vi "Material-ConfigDialog-UI.vi"(11 "error in":errorcluster) -> (15 "error out":errorcluster)   [LabVIEW 2014, in "Material-ConfigDialog.lvclass"]
uses:
  Material-ConfigDialog.lvclass
  Reuse Library/featherweight/Core/Sequencer/FTW-Sequencer.lvclass/FTW-Sequencer.ctl
  Material-ConfigDialog-Page.ctl
  Reuse Library/featherweight/Core/Messaging/Messenger.Actor/FTW-Messenger-Actor.lvclass
  Material-ConfigDialog.lvclass/Material-ConfigDialog.ctl
  <instrlib>/Keyence LK-G5000/Public/Constant/Comm Interface.ctl
  <vilib>/Utility/error.llb/DialogType.ctl
  Glue/Material-Glue-TreeItem.ctl
  Reuse Library/featherweight/Core/Regex/FTW-Regex.vi
  Reuse Library/featherweight/Core/Error/FTW-ERR-StatusException.vi
  Reuse Library/featherweight/Core/Error/FTW-ERR-ThrowError.vi
  Reuse Library/featherweight/Core/Error/FTW-ERR-Clear.vi
  Deploy Application/Material-Application-Constants.vi
  Reuse Library/featherweight/Core/Sequencer/FTW-Sequencer.lvclass
  Reuse Library/featherweight/Core/Messaging/Message.Actor/FTW-Message-Actor.lvclass
  Automation/Material-Automation-Website.ctl
  <instrlib>/Keyence LK-G5000/Keyence LK-G5000.lvlib
  <resource>/Framework/Providers/Wirebird Labs LLC/Deploy/Support/Update Service/Deploy-UpdateService.lvclass
panel:
  in  "UI_Tree_Navigation":string(tree) caption="Navigation Tree"
  in  "Hidden Controls\n(Tab Control Container)":enum32{"Just some hidden controls"}(tab)
  out "Status Bar Messages":string
  in  "UI-Button-Save":bool caption="Save Button"
  in  "UI-Button-Cancel":bool caption="Cancel Button"
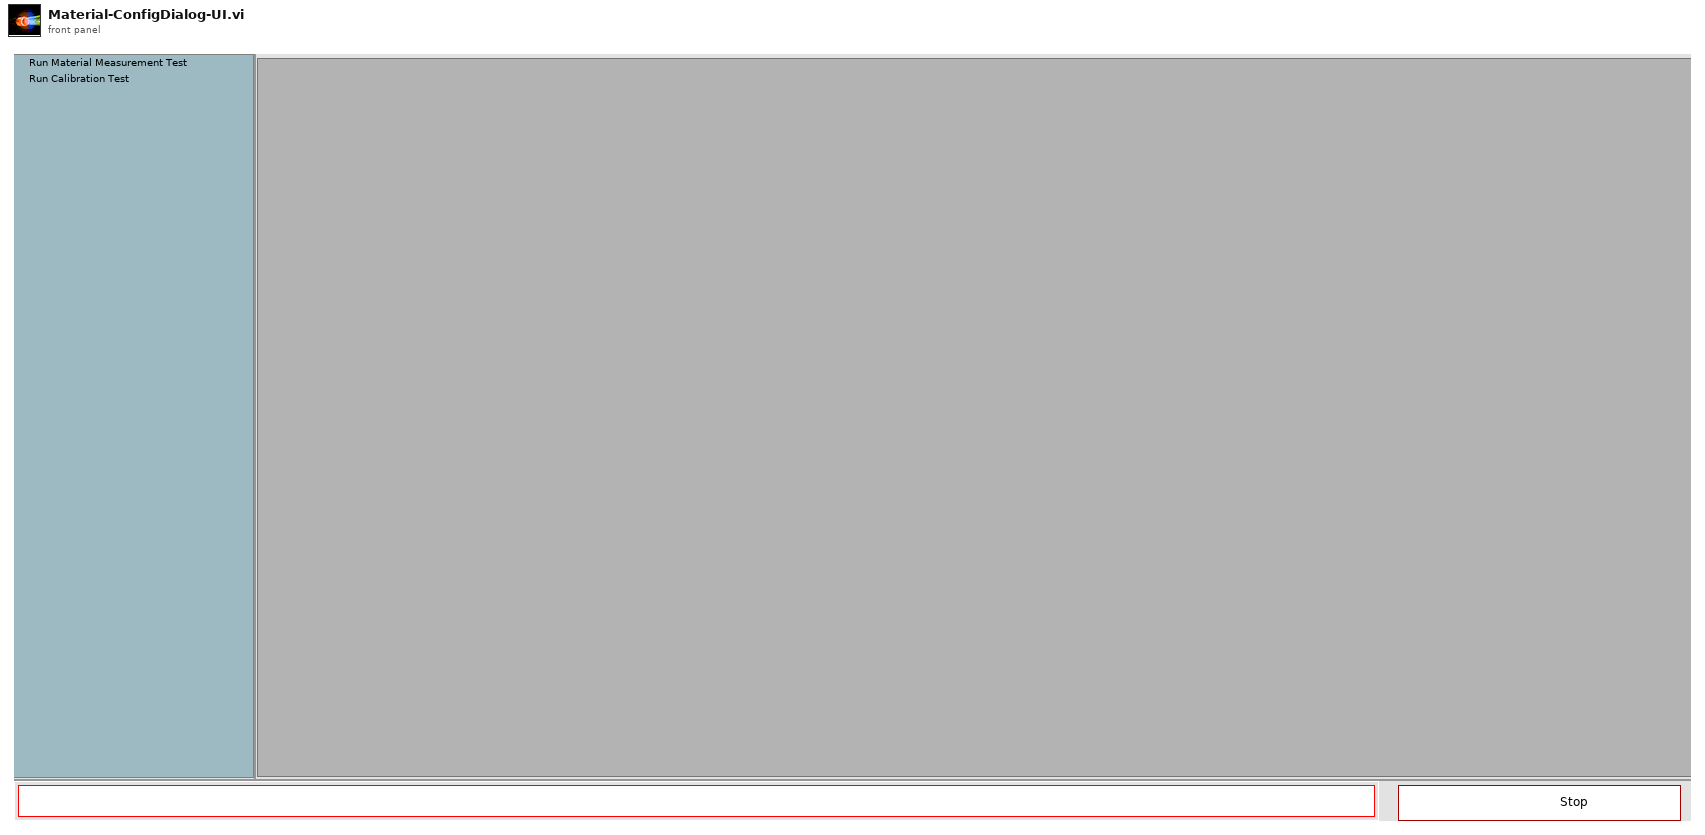
[diagram p1: front panel]
types:
  T1 = typedef "Material-Automation-Website.ctl" = enum16{"Wirebird Labs Home", "Wirebird Labs Support Home", "Wirebird Labs Licensing", "Wirebird Labs Idea Exchange", "Wirebird Labs Report a Bug", "Wirebird Labs Services Status", "Contact Wirebird Labs", "Deploy Documentation", "Deploy Credits", "Deploy Marketing", "Deploy Feature Matrix", "Deploy Purchase", "Deploy Deployment Servers"}
  T2 = typedef "Keyence LK-G5000.lvlib/Comm Interface.ctl" = enum8{"USB", "ETHERNET"}
  T3 = typedef "Material-Glue-TreeItem.ctl" = cluster{"Tag":string, "Parent":string, "Add to Top of Parent":bool, "Type":string, "Indent":i32, "Child Only":bool, "First Cell":string, "Next Cells":string[]}
  T4 = typedef "Material-ConfigDialog.lvclass/Material-ConfigDialog-Page.ctl" = cluster{"Initialized?":bool, "PageID":string, "Messenger":refnum<class "FTW-Messenger-Actor.lvclass">}
  T5 = cluster{"Configuration Dialog Mailbox":refnum<event-registration>, "Update Service Event Registration":refnum<event-registration>}
  T6 = typedef "DialogType.ctl" = u16
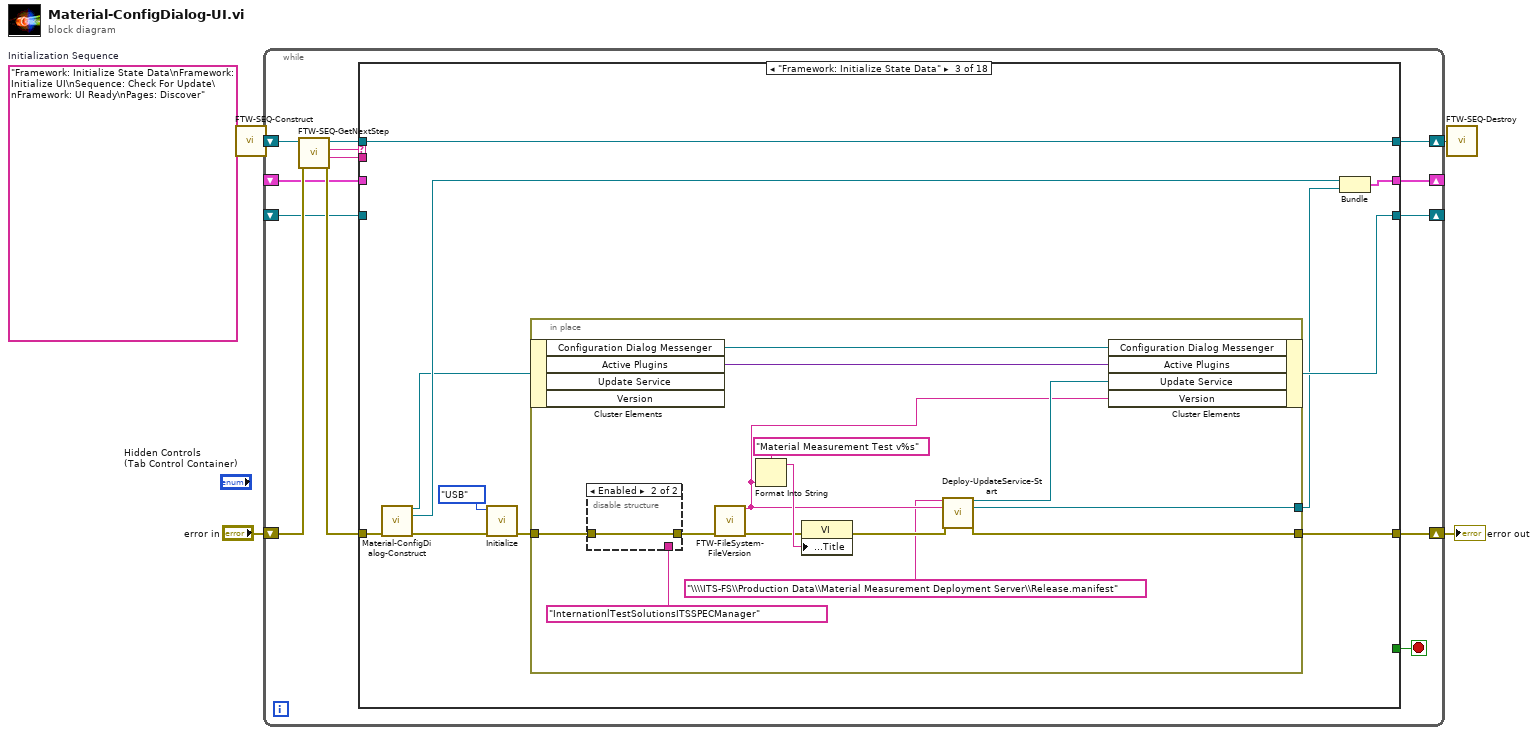
[diagram p0: block diagram]
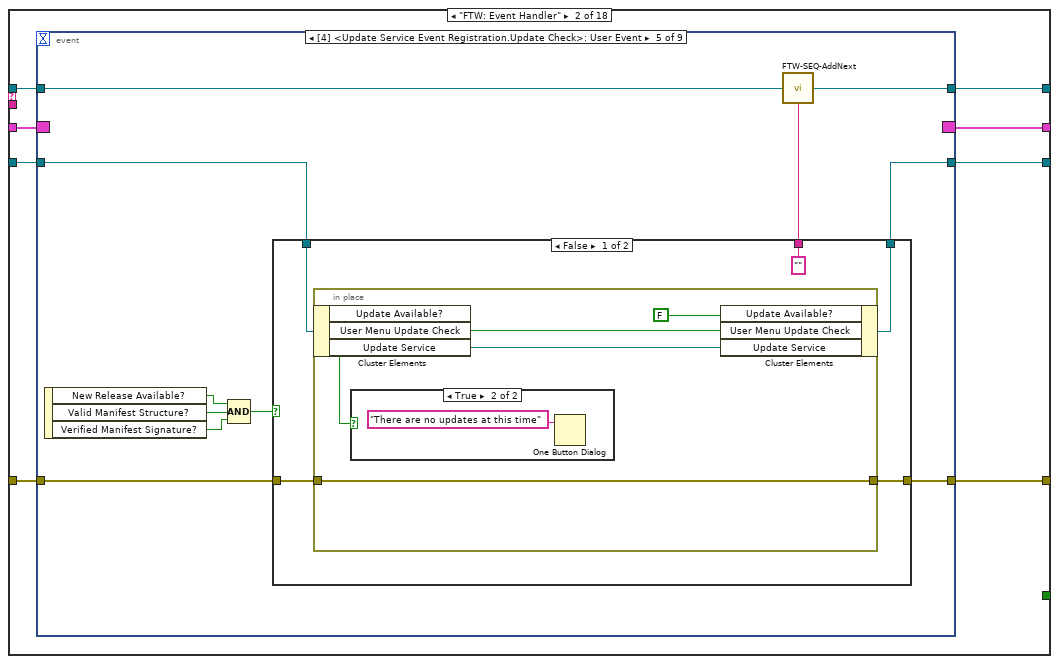
[diagram p3: hidden frame]
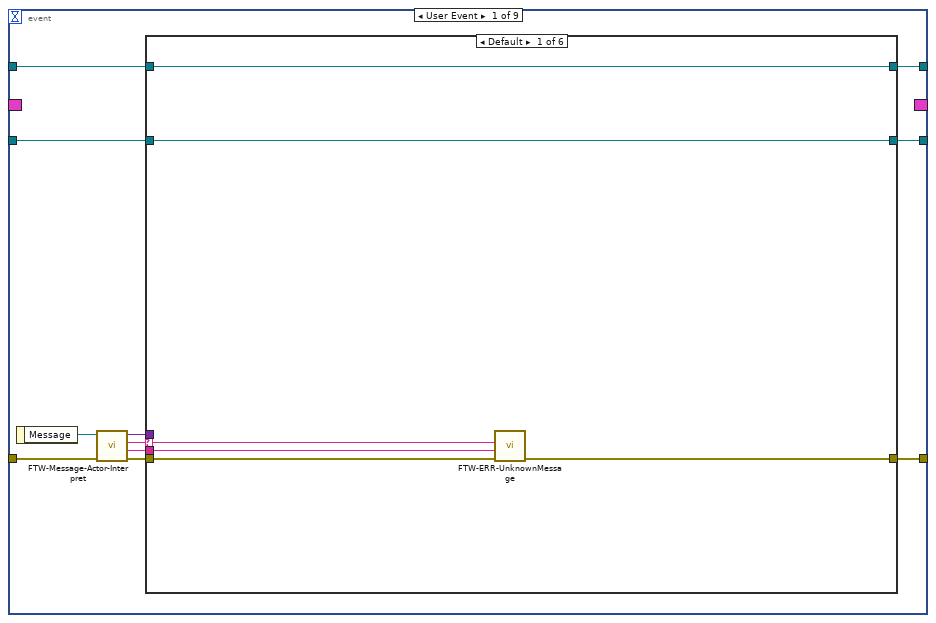
[diagram p4: hidden frame]
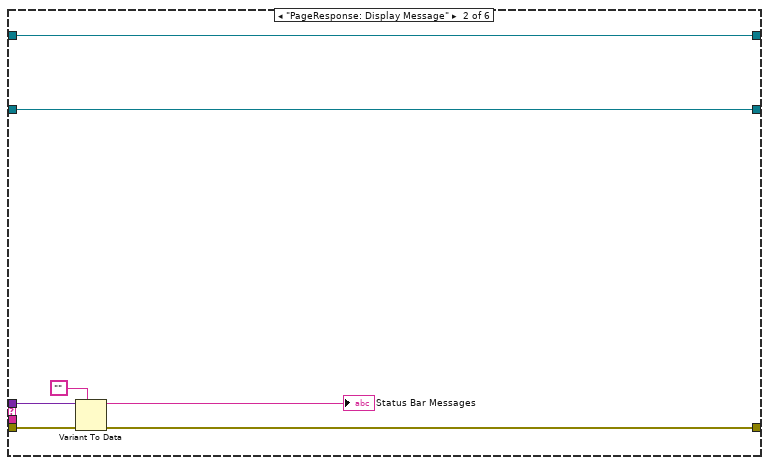
[diagram p5: hidden frame]
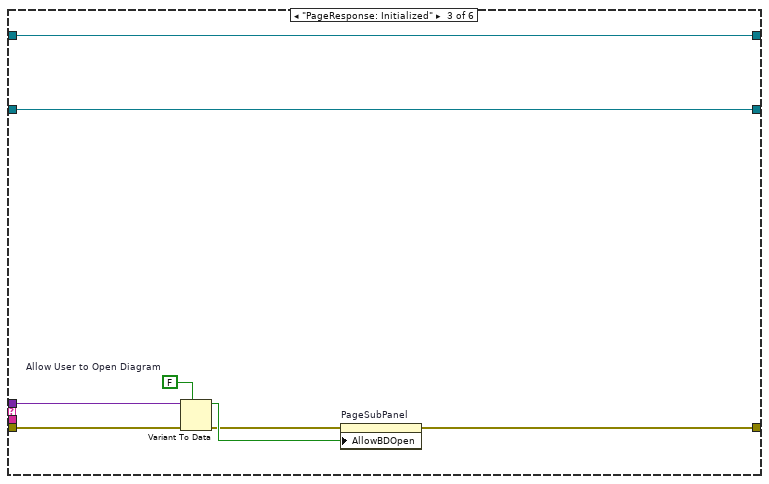
[diagram p6: hidden frame]
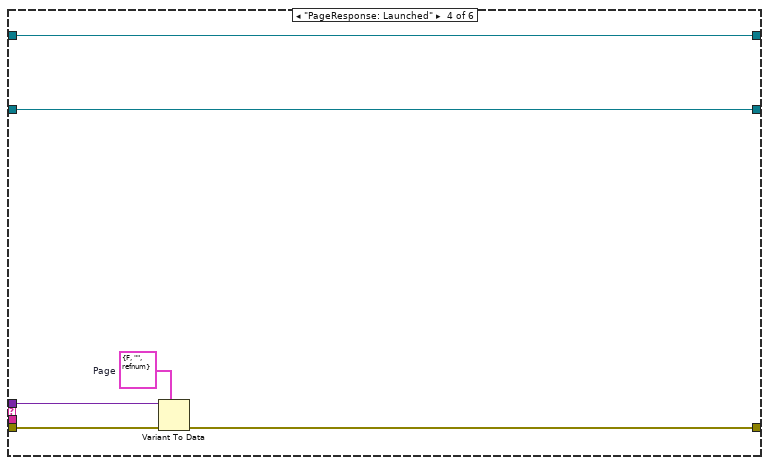
[diagram p7: hidden frame]
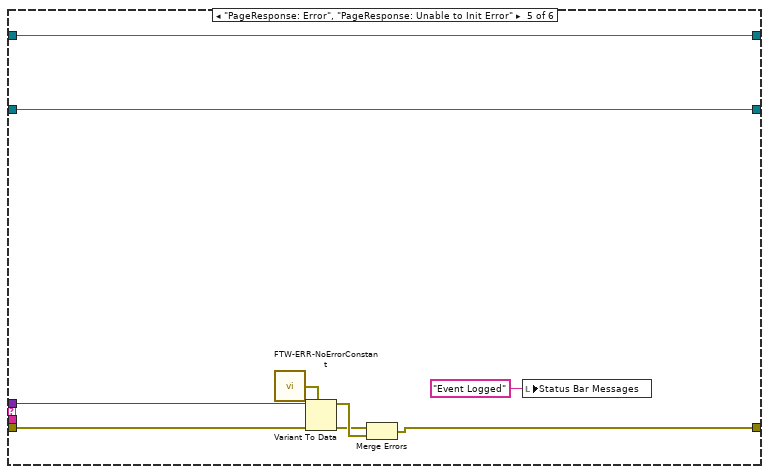
[diagram p8: hidden frame]
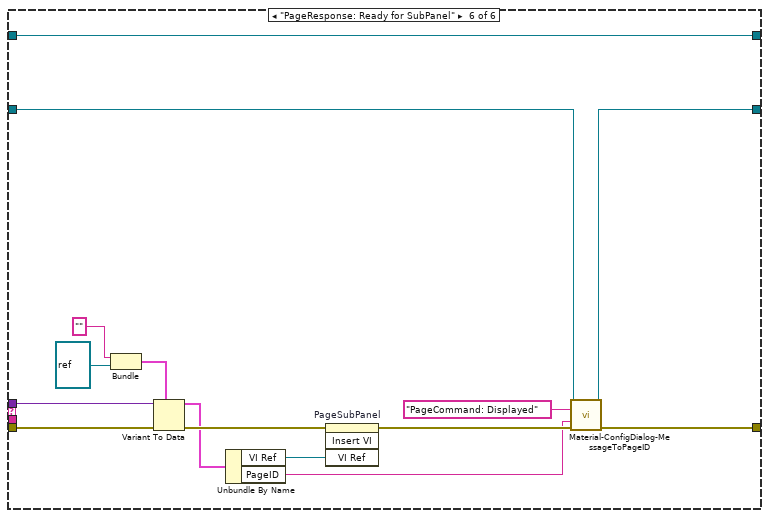
[diagram p9: hidden frame]
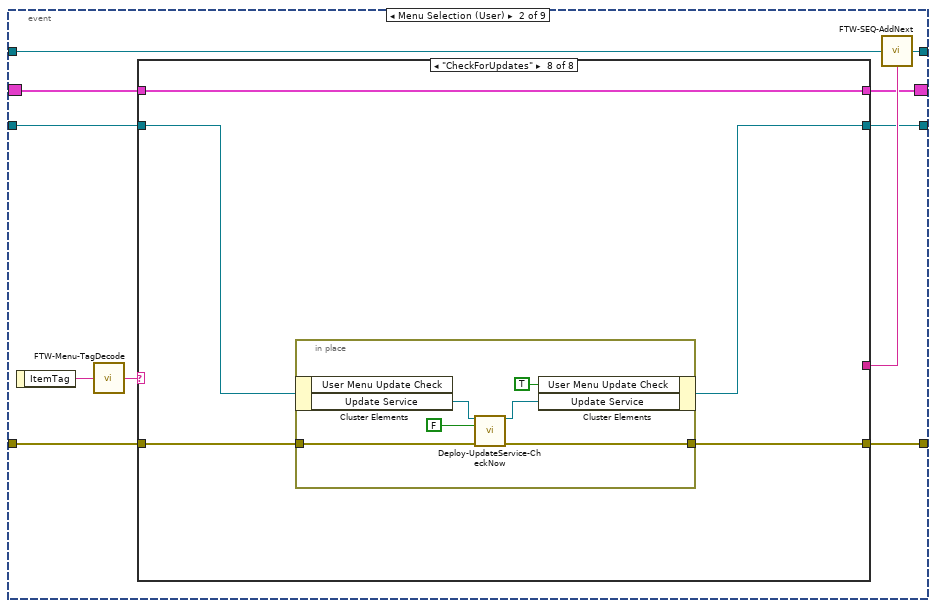
[diagram p10: hidden frame]
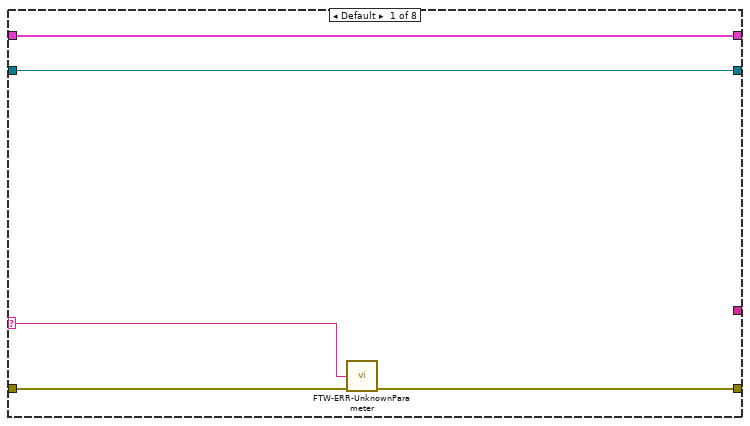
[diagram p11: hidden frame]
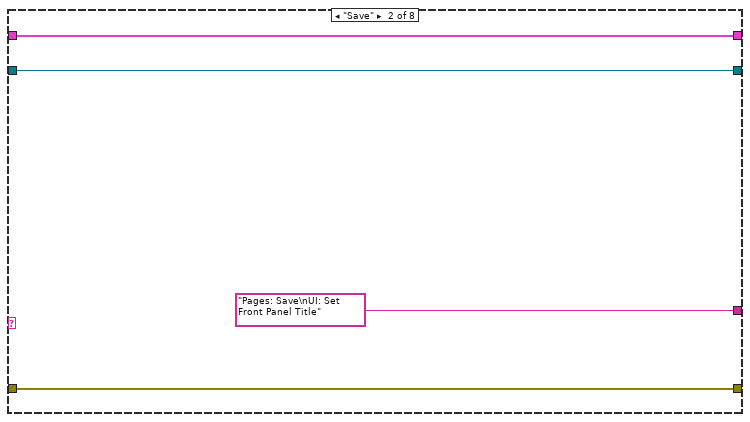
[diagram p12: hidden frame]
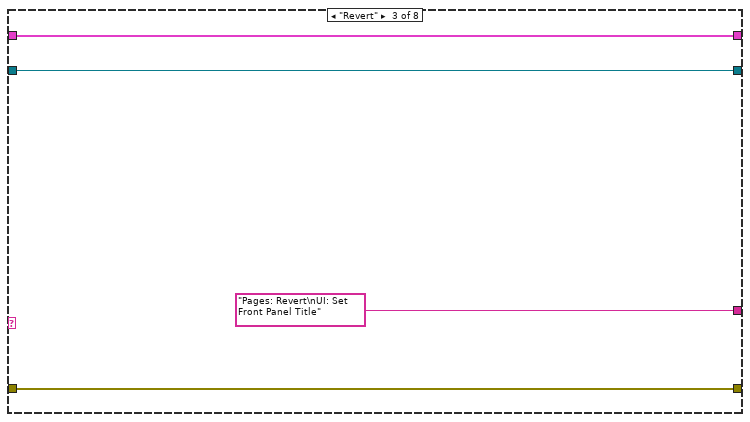
[diagram p13: hidden frame]
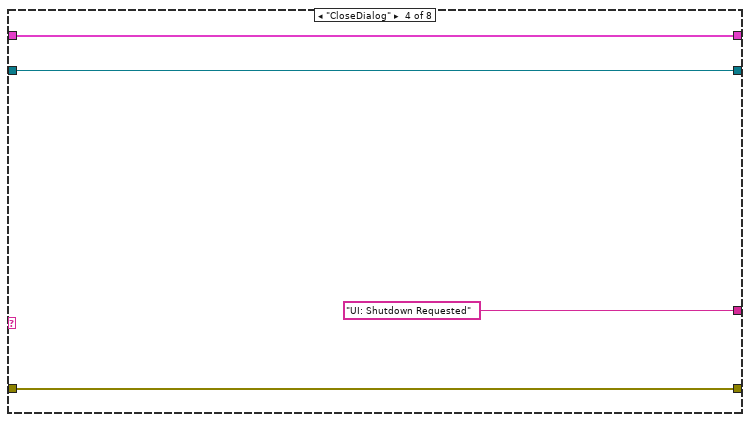
[diagram p14: hidden frame]
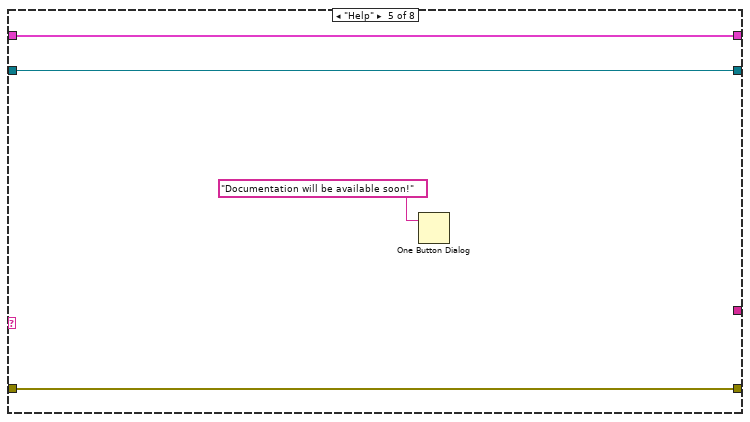
[diagram p15: hidden frame]
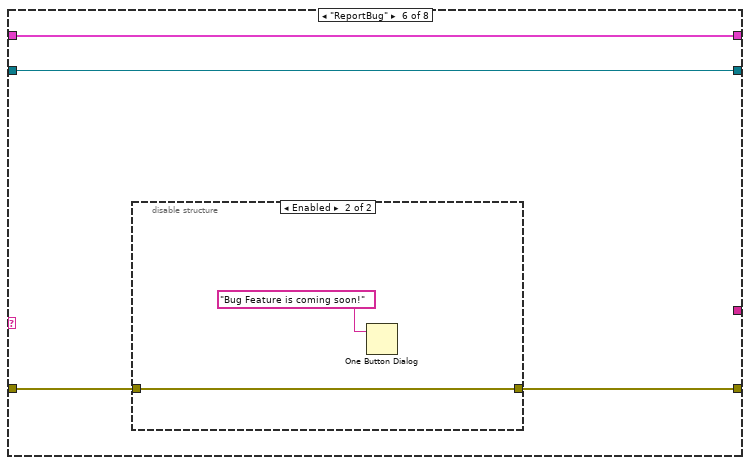
[diagram p16: hidden frame]
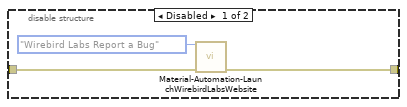
[diagram p17: hidden frame]
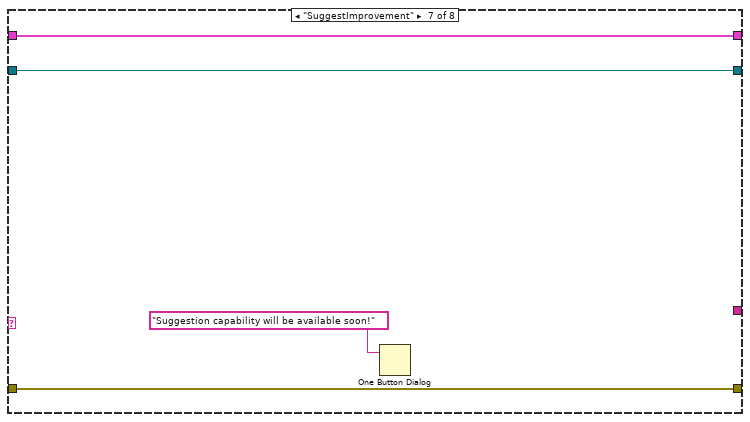
[diagram p18: hidden frame]
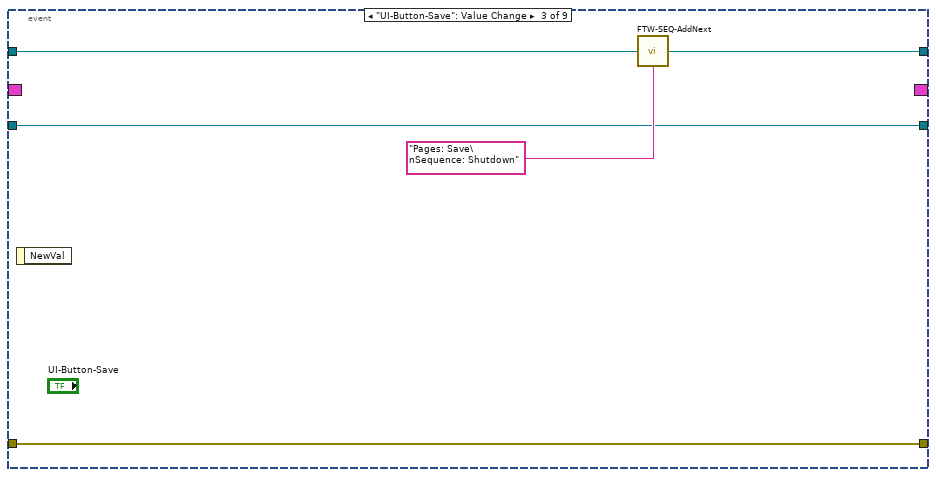
[diagram p19: hidden frame]
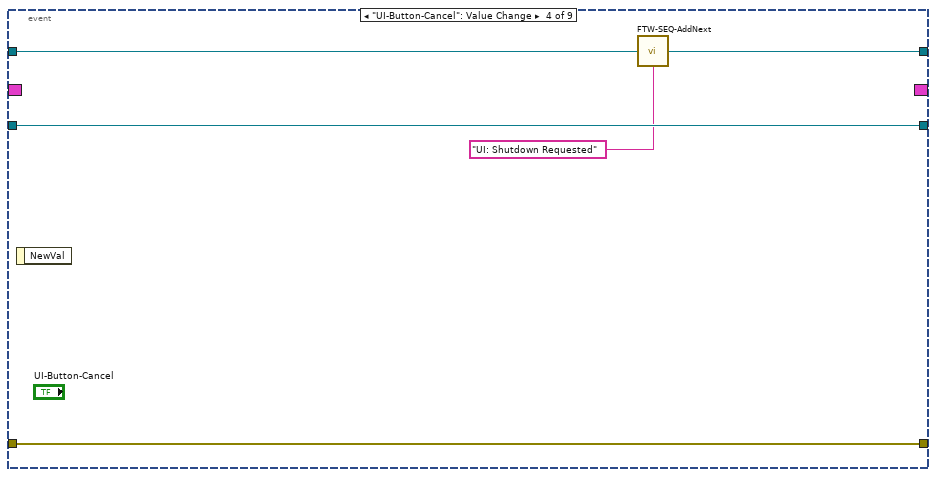
[diagram p20: hidden frame]
diagram:
  w5 = "Framework: Initialize State Data\nFramework: Initialize UI\nSequence: Check For Update\nFramework: UI Ready\nPages: Discover"  # Initialization Sequence
  n1 = call "FTW-SEQ-Construct.vi"("Initial Sequence"=w5) -> ("Sequencer"=w2:refnum<class "FTW-Sequencer.lvclass">)
  n2 = while {
    shift-right: [w16] -> w1
    shift-left: w2 -> [w7]
    shift-right: [w17] -> w4
    shift-left: "error in" -> [w15]
    shift-right: [w10] -> _
    shift-left: _ -> [w11]
    shift-right: [w9] -> _
    shift-left: _ -> [w8]
    stop <- w12 stop-if-true
    n3 = call "FTW-SEQ-GetNextStep.vi"("error in"=w15, "Sequencer"=w7) -> ("error out"=w18:errorcluster, "Job Data"=w6:string, "Current Job"=w13:string, "Sequencer out"=w14:refnum<class "FTW-Sequencer.lvclass">)  [unwired: 6 in]
    n4 = case shown="\"Framework: Initialize State Data\"" w13 {
      selector: w13 -> [_ _ _ _ _ _ w330 _ _ _ _ _ _ _ _ _ _ _]
      tunnel: [w20 w28 w258 w294 w318 w326 w332 w352 w353 w361 w367 w372 w393 w395 w411 w432 w445 w454] -> w17
      tunnel: w18 -> [w20 w27 w262 w295 w319 w324 w333 w348 w354 w361 w367 w373 w393 w395 w411 w420 w441 w449]
      tunnel: w14 -> [w22 w30 w261 w316 w322 w329 w335 w351 w359 w363 w364 w374 w392 w399 w412 w435 w448 w456]
      tunnel: [w22 w29 w261 w316 w322 w329 w335 w351 w359 w363 w369 w374 w392 w401 w412 w435 w448 w456] -> w16
      tunnel: [_ _ _ _ _ _ _ _ TRUE _ _ _ _ _ _ _ _ _] -> w12
      tunnel: w11 -> [w21 w25 _ w315 w321 w328 w334 w346 w357 w362 w368 w375 w394 w402 w414 w434 w447 w455]
      tunnel: [w21 w26 w263 w315 w321 w328 w334 w346 w357 w362 w368 w375 w394 w402 w414 w434 w447 w455] -> w10
      tunnel: [w19 w24 w257 w314 w320 w327 w331 w337 w356 w360 w365 w370 w391 w400 w413 w421 w446 w453] -> w9
      tunnel: w8 -> [w19 w23 _ w314 w320 w327 w331 w337 w356 w360 w365 w371 w391 w400 w413 w421 w442 w450]
      tunnel: w6 -> [_ _ _ _ _ _ _ _ _ _ _ _ _ _ _ _ _ _]
      frame "--------- Framework ---------" {
      }
      frame "FTW: Event Handler" {
        n5 = event shown="[4] <Update Service Event Registration.Update Check>: User Event" {
          selector: w25 -> [_ w93 _ _ _ _ _ _ _]
          dyn-events: [_ w94 _ _ _ _ _ _ _] -> w26
          timeout: _ -> [_ _ _ _ _ _ _ _ _]
          tunnel: w30 -> [w34 w99 w149 w155 w161 w204 w222 w244 w248]
          tunnel: [w35 w103 w153 w158 w163 w204 w222 w244 w251] -> w29
          tunnel: [w38 w100 w152 w156 w160 w209 w223 w245 w252] -> w28
          tunnel: w27 -> [w39 w101 w152 w156 w159 w210 w219 w246 w252]
          tunnel: [w37 w96 w150 w157 w164 w205 w221 w243 w249] -> w24
          tunnel: w23 -> [w36 w95 w150 w157 w165 w205 w216 w243 w249]
          event User Event {
            n6 = event-data() -> ("Message"=w40:refnum<class "FTW-Message.lvclass">)  [unwired: 1 in]
            n7 = call "FTW-Message-Actor-Interpret.vi"("error in"=w39, "Message"=w40) -> ("error out"=w41:errorcluster, "Sender"=w31:string, "Parameter"=w33:string, "Payload"=w32:variant)  [unwired: 6 in]
            n8 = case shown="Default" w33 {
              selector: w33 -> [w43 _ _ _ _ _]
              tunnel: w32 -> [_ w54 w55 w65 w77 w92]
              tunnel: [w46 w52 w56 w63 w69 w85] -> w38
              tunnel: w41 -> [w47 w53 w60 w64 w76 w91]
              tunnel: [w44 w48 w62 w68 w73 w87] -> w37
              tunnel: w36 -> [w44 w48 w62 w68 w73 w88]
              tunnel: [w45 w49 w61 w67 w74 w90] -> w35
              tunnel: w34 -> [w45 w49 w61 w67 w74 w90]
              tunnel: w31 -> [w42 _ _ _ _ _]
              frame Default {
                n9 = call "FTW-ERR-UnknownMessage.vi"("error in"=w47, "Sender"=w42, "Unknown Parameter"=w43) -> ("error out"=w46:errorcluster)  [unwired: 8 in]
              }
              frame "PageResponse: Display Message" {
                n10 = Variant To Data(error in=w53, type="", Variant=w54) -> (data=→"Status Bar Messages":string, error out=w52:errorcluster)
              }
              frame "PageResponse: Initialized" {
                w59 = FALSE  # Allow User to Open Diagram
                n11 = Variant To Data(error in=w60, type=w59, Variant=w55) -> (data=w58:bool, error out=w57:errorcluster)
                n12 = property on="PageSubPanel" class="SubPnl"(error in=w57, "AllowBDOpen"=w58) -> (error out=w56:errorcluster)  [unwired: 1 in, 1 out]
              }
              frame "PageResponse: Launched" {
                w66 = T4 {"Initialized?"=FALSE, "PageID"="", "Messenger"=refnum}  # Page
                n13 = Variant To Data(error in=w64, type=w66, Variant=w65) -> (error out=w63:errorcluster)  [unwired: 1 out]
              }
              frame "PageResponse: Error", "PageResponse: Unable to Init Error" {
                n14 = call "FTW-ERR-NoErrorConstant.vi"() -> ("no error"=w75:errorcluster)
                n15 = Variant To Data(error in=w76, type=w75, Variant=w77) -> (data=w71:errorcluster, error out=w70:errorcluster)
                n16 = Merge Errors(w70, w71) -> (w69:errorcluster)
                n17 = local write "Status Bar Messages"("Event Logged" ("Status Bar Messages")) -> ()
              }
              frame "PageResponse: Ready for SubPanel" {
                n18 = Bundle("PageID"="", "VI Ref"=refnum<vi> refnum) -> (w81:cluster{"PageID":string, "VI Ref":refnum<vi>})  [unwired: 1 in]
                n19 = Variant To Data(error in=w91, type=w81, Variant=w92) -> (data=w80:cluster{"PageID":string, "VI Ref":refnum<vi>}, error out=w84:errorcluster)
                n20 = Unbundle By Name(w80) -> ("VI Ref"=w79:refnum<vi>, "PageID"=w78:string)
                n21 = invoke on="PageSubPanel" class="SubPanel" method="Insert VI"(error in=w84, "VI Ref"=w79) -> (error out=w86:errorcluster)  [unwired: 2 in, 3 out]
                n22 = call "Material-ConfigDialog-MessageToPageID.vi"("Configuration Dialog"=w88, "Parameter"="PageCommand: Displayed", "PageID"=w78, "error in"=w86) -> ("Configuration Dialog out"=w87:refnum<class "Material-ConfigDialog.lvclass">, "error out"=w85:errorcluster)  [unwired: 10 in]
              }
            }
          }
          event Menu Selection (User) {
            n23 = event-data() -> ("ItemTag"=w98:string)  [unwired: 1 in]
            n24 = call "FTW-Menu-TagDecode.vi"("Menu Item Tag"=w98) -> ("Command"=w97:string)  [unwired: 1 in, 2 out]
            n25 = case shown="\"CheckForUpdates\"" w97 {
              selector: w97 -> [w105 _ _ _ _ _ _ _]
              tunnel: [_ "Pages: Save\nUI: Set Front Panel Title" ("Add to Top of Queue") "Pages: Revert\nUI: Set Front Panel Title" ("Add to Top of Queue") "UI: Shutdown Requested" ("Add to Top of Queue") _ _ _ _] -> w102
              tunnel: w101 -> [w108 w111 w115 w119 w124 w128 w135 w141]
              tunnel: [w107 w111 w115 w119 w124 w127 w135 w140] -> w100
              tunnel: [w106 w110 w114 w118 w123 w126 w137 w138] -> w96
              tunnel: w95 -> [w106 w110 w114 w118 w123 w126 w137 w139]
              tunnel: [w104 w109 w113 w117 w122 w125 w136 w142] -> w94
              tunnel: w93 -> [w104 w109 w113 w117 w122 w125 w136 w142]
              frame Default {
                n26 = call "FTW-ERR-UnknownParameter.vi"("Unknown Parameter"=w105, "error in"=w108) -> ("error out"=w107:errorcluster)  [unwired: 13 in]
              }
              frame "Save" {
              }
              frame "Revert" {
              }
              frame "CloseDialog" {
              }
              frame "Help" {
                n27 = One Button Dialog(message="Documentation will be available soon!") -> ()  [unwired: 1 in, 1 out]
              }
              frame "ReportBug" {
                n28 = disable-structure shown="Enabled" {
                  disable-tunnel: w128 -> [w131 w133]
                  disable-tunnel: [w130 w133] -> w127
                  frame Disabled {
                    n29 = call "Material-Automation-LaunchWirebirdLabsWebsite.vi"("Site to Launch"=Material-Automation-Website."Wirebird Labs Report a Bug", "error in"=w131) -> ("error out"=w130:errorcluster)  [unwired: 13 in]
                  }
                  frame Enabled {
                    n30 = One Button Dialog(message="Bug Feature is coming soon!") -> ()  [unwired: 1 in, 1 out]
                  }
                }
              }
              frame "SuggestImprovement" {
                n31 = One Button Dialog(message="Suggestion capability will be available soon!") -> ()  [unwired: 1 in, 1 out]
              }
              frame "CheckForUpdates" {
                n32 = in-place {
                  in-place-border: w141 -> [w148]
                  in-place-border: [w144] -> w140
                  n33 = in-place-cluster #1(w139) -> ("Update Service"=w146:refnum<class "Deploy-UpdateService.lvclass">)  [unwired: 1 out]
                  n34 = call <resource>:"Deploy-UpdateService-CheckNow.vi"("Update Service"=w146, "Show UI?"=FALSE, "error in"=w148) -> ("Update Service out"=w145:refnum<class "Deploy-UpdateService.lvclass">, "error out"=w144:errorcluster)  [unwired: 11 in]
                  n35 = in-place-cluster #1("User Menu Update Check"=TRUE, "Update Service"=w145) -> (w138:refnum<class "Material-ConfigDialog.lvclass">)
                }
              }
            }
            n36 = call "FTW-SEQ-AddNext.vi"("Add Next in Sequence"=w102, "Sequencer"=w99) -> ("Sequencer out"=w103:refnum<class "FTW-Sequencer.lvclass">)  [unwired: 2 in]
          }
          event "UI-Button-Save": Value Change {
            n37 = event-data() -> ()  [unwired: 1 in, 1 out]
            n38 = call "FTW-SEQ-AddNext.vi"("Add Next in Sequence"="Pages: Save\nSequence: Shutdown" ("Add to Top of Queue"), "Sequencer"=w149) -> ("Sequencer out"=w153:refnum<class "FTW-Sequencer.lvclass">)  [unwired: 2 in]
          }
          event "UI-Button-Cancel": Value Change {
            n39 = event-data() -> ()  [unwired: 1 in, 1 out]
            n40 = call "FTW-SEQ-AddNext.vi"("Add Next in Sequence"="UI: Shutdown Requested" ("Add to Top of Queue"), "Sequencer"=w155) -> ("Sequencer out"=w158:refnum<class "FTW-Sequencer.lvclass">)  [unwired: 2 in]
          }
          event User Event {
            n41 = event-data() -> ("New Release Available?"=w169:bool, "Valid Manifest Structure?"=w168:bool, "Verified Manifest Signature?"=w167:bool)  [unwired: 1 in]
            n42 = Compound Arithmetic op=AND(w169, w168, w167) -> (w166:bool)
            n43 = case shown="False" w166 {
              selector: w166 -> [_ w182]
              tunnel: w159 -> [w172 w185]
              tunnel: w165 -> [w173 w183]
              tunnel: [w170 w181] -> w164
              tunnel: [w171 w184] -> w160
              tunnel: ["" ("Application Shutdown") w180] -> w162
              frame False {
                n44 = in-place {
                  in-place-border: w172 -> [w175]
                  in-place-border: [w175] -> w171
                  n45 = in-place-cluster #2(w173) -> ("User Menu Update Check"=w178:bool, "Update Service"=w176:refnum<class "Deploy-UpdateService.lvclass">)  [unwired: 1 out]
                  n46 = case shown="True" w178 {
                    frame False {
                    }
                    frame True {
                      n47 = One Button Dialog(message="There are no updates at this time" ("Application Shutdown")) -> ()  [unwired: 1 in, 1 out]
                    }
                  }
                  n48 = in-place-cluster #2("Update Available?"=FALSE, "User Menu Update Check"=w178, "Update Service"=w176) -> (w170:refnum<class "Material-ConfigDialog.lvclass">)
                }
              }
              frame True {
                n49 = in-place {
                  in-place-border: w185 -> [w195]
                  in-place-border: [w190] -> w184
                  in-place-border: w182 -> [_]
                  in-place-border: [w186] -> w180
                  n50 = in-place-cluster #3(w183) -> ("Update Service"=w194:refnum<class "Deploy-UpdateService.lvclass">, "Version"=w188:string)  [unwired: 1 out]
                  n51 = call <resource>:"Deploy-UpdateService-Stop.vi"("Update Service"=w194, "error in"=w195) -> ("error out"=w192:errorcluster)  [unwired: 13 in]
                  n52 = Equal?(x=w188, y="IDE") -> (x = y?=w189:bool)
                  n53 = case shown="True" w189 {
                    tunnel: w192 -> [w201 w203]
                    tunnel: "\\\\ITS-FS\\Production Data\\Material Measurement Deployment Server\\Release.manifest" ("Manifest URI") -> [w200 _]
                    tunnel: [w198 w203] -> w190
                    tunnel: w188 -> [w197 _]
                    tunnel: [w196 "" ("Application Shutdown")] -> w186
                    frame False {
                      w196 = "Sequence: Shutdown"  # Application Shutdown
                      n54 = call <resource>:"Deploy-UpdateService-LaunchUI-Async.vi"("Manifest URI"=w200, "Current Release Version"=w197, "error in"=w201, "Installer Command Line Parameters"="") -> ("error out"=w198:errorcluster)  [unwired: 10 in, 1 out]
                    }
                    frame True {
                    }
                  }
                  n55 = in-place-cluster #3("Update Service"=w194, "Update Available?"=TRUE ("Boolean"), "Version"=w188) -> (w181:refnum<class "Material-ConfigDialog.lvclass">)
                }
              }
            }
            n56 = call "FTW-SEQ-AddNext.vi"("Add Next in Sequence"=w162, "Sequencer"=w161) -> ("Sequencer out"=w163:refnum<class "FTW-Sequencer.lvclass">)  [unwired: 2 in]
          }
          event User Event {
            n57 = event-data() -> ("Error Status"=w208:bool, "Error Code"=w207:i32, "Error Message"=w206:string)  [unwired: 1 in]
            n58 = Format Into String(format string="Uh-oh! Something went wrong! This is what happened:\n\nError %d: \"%s\"", w207, w206) -> (resulting string=w212:string)  [unwired: 2 in, 1 out]
            n59 = One Button Dialog(message=w212) -> ()  [unwired: 1 in, 1 out]
            n60 = Bundle By Name(cluster=w210, "status"=w208, "code"=w207, "source"=w206) -> (w209:errorcluster)
          }
          event "UI_Tree_Navigation": Value Change {
            n61 = event-data() -> ("NewVal"=w214:string)  [unwired: 1 in]
            n62 = call "FTW-Menu-TagDecode.vi"("Menu Item Tag"=w214) -> ("Command"=w220:string, "Payload"=w217:string)  [unwired: 1 in, 1 out]
            n63 = case shown="\"UninitializedPage\"" w220 {
              tunnel: w219 -> [w227 w231 w242]
              tunnel: [w226 w231 w233] -> w218
              tunnel: w217 -> [_ _ w241]
              tunnel: w216 -> [w225 w230 w239]
              tunnel: [w225 w230 w238] -> w215
              tunnel: w214 -> [_ _ w236]
              tunnel: [_ "UI_Tree_Navigation" w235] -> w213
              frame Default {
                n64 = call "FTW-ERR-ThrowGenericError.vi"("Error Message"="Unknown Navigation Tree item.", "error in"=w227) -> ("error out"=w226:errorcluster)  [unwired: 13 in]
              }
              frame "ActivePage" {
                # "Already launched; just notify it\nneeds to get ready for SubPanel"
              }
              frame "UninitializedPage" {
                # "Keep\nselection"
                n65 = String To Path(string=w241) -> (path=w240:path)
                n66 = call "Material-ConfigDialog-LaunchPage.vi"("Configuration Dialog"=w239, "Configuration Page VI Filepath"=w240, "error in"=w242) -> ("Configuration Dialog out"=w238:refnum<class "Material-ConfigDialog.lvclass">, "New Navigation Tree Tag"=w235:string, "error out"=w237:errorcluster)  [unwired: 9 in, 1 out]
                n67 = invoke on="UI_Tree_Navigation" class="Tree (strict)" method="Edit Tree Items.Set Tag"(error in=w237, "tag"=w236, "new tag"=w235) -> (error out=w234:errorcluster, "Edit Tree Items:Set Tag"=w232:string)  [unwired: 2 in, 3 out]
                n68 = property on="UI_Tree_Navigation" class="Tree (strict)"(error in=w234, "Value"=w232) -> (error out=w233:errorcluster)  [unwired: 1 in, 1 out]
              }
            }
            n69 = call "Material-ConfigDialog-MessageToPageID.vi"("Configuration Dialog"=w215, "Parameter"="PageCommand: Prepare for SubPanel", "PageID"=w213, "error in"=w218) -> ("Configuration Dialog out"=w221:refnum<class "Material-ConfigDialog.lvclass">, "error out"=w223:errorcluster)  [unwired: 10 in]
          }
          event "UI_Tree_Navigation": Mouse Down {
            # "Just ensure the pesky dotted box\nsurrounding the item does not show up"
            n70 = event-data() -> ()  [unwired: 1 in, 2 out]
            n71 = property on="UI_Tree_Navigation" class="Tree (strict)"(error in=w246, "Key Focus"=FALSE) -> (error out=w245:errorcluster)  [unwired: 1 in, 1 out]
          }
          event Panel Close? {
            n72 = event-data() -> ()  [unwired: 1 in, 1 out]
            n73 = call "FTW-SEQ-AddNext.vi"("Add Next in Sequence"="UI: Shutdown Requested" ("Add to Top of Queue"), "Sequencer"=w248) -> ("Sequencer out"=w251:refnum<class "FTW-Sequencer.lvclass">)  [unwired: 2 in]
            n74 = event-data("Discard?"=TRUE) -> ()  [unwired: 1 in, 1 out]
          }
        }
      }
      frame "Framework: Initialize State Data" {
        n75 = call "Material-ConfigDialog-Construct.vi"("error in"=w262) -> ("Configuration Dialog"=w259:refnum<class "Material-ConfigDialog.lvclass">, "Configuration Dialog Mailbox"=w264:refnum<event-registration>, "error out"=w255:errorcluster)  [unwired: 12 in]
        n76 = call <instrlib>:"Initialize.vi"("error in (no error)"=w255, "Comm Interface"=Comm_Interface."USB") -> ("error out"=w254:errorcluster)  [unwired: 9 in]
        n77 = in-place {
          in-place-border: [w278] -> w256
          in-place-border: [w274] -> w258
          in-place-border: w254 -> [w265]
          n78 = in-place-cluster #4(w259) -> ("Configuration Dialog Messenger"=w275:refnum<class "FTW-Messenger-Actor.lvclass">, "Active Plugins"=w276:variant)  [unwired: 2 out]
          n79 = disable-structure shown="Enabled" {
            disable-tunnel: w265 -> [w281 w282]
            disable-tunnel: [w280 w282] -> w269
            disable-tunnel: "InternationlTestSolutionsITSSPECManager" ("format string") -> [w279 _]
            frame Disabled {
              n80 = call <resource>:"Deploy-Update-CreateAppMutex.vi"("Application Mutex Name"=w279, "error in"=w281) -> ("error out"=w280:errorcluster)  [unwired: 13 in]
            }
            frame Enabled {
            }
          }
          n81 = call "FTW-FileSystem-FileVersion.vi"("error in"=w269) -> ("Version"=w268:string, "error out"=w271:errorcluster)  [unwired: 13 in]
          n82 = Format Into String(format string="Material Measurement Test v%s", w268) -> (resulting string=w272:string)  [unwired: 2 in, 1 out]
          n83 = property class="VI"(error in=w271, "Front Panel.Title"=w272) -> (error out=w270:errorcluster)  [unwired: 1 in, 1 out]
          n84 = call <resource>:"Deploy-UpdateService-Start.vi"("Manifest URI"="\\\\ITS-FS\\Production Data\\Material Measurement Deployment Server\\Release.manifest", "Current Release Version"=w268, "error in"=w270) -> ("Update Service"=w277:refnum<class "Deploy-UpdateService.lvclass">, "Update Service Event Registration"=w278:refnum<event-registration>, "error out"=w274:errorcluster)  [unwired: 10 in]
          n85 = in-place-cluster #4("Configuration Dialog Messenger"=w275, "Active Plugins"=w276, "Update Service"=w277, "Version"=w268) -> (w257:refnum<class "Material-ConfigDialog.lvclass">)
        }
        n86 = Bundle("Configuration Dialog Mailbox"=w264, "Update Service Event Registration"=w256) -> (w263:T5)  [unwired: 1 in]
      }
      frame "Framework: Initialize UI" {
        w297 = i16 40 ("Vertical")
        w300 = i16 240 ("Horizontal")
        w306 = 2000  # Much wider than ever expected to be
        n87 = invoke on="UI_Tree_Navigation" class="Tree (strict)" method="Edit Tree Items.Delete"("Delete Children"=TRUE ("Delete Children?")) -> (error out=w291:errorcluster)  [unwired: 4 in, 4 out]
        n88 = call "Material-Application-MinimumPageSize.vi"("error in"=w295) -> ("Minimum Pane Size"=w290:cluster{"Horizontal":i16, "Vertical":i16}, "error out"=w305:errorcluster)  [unwired: 13 in]
        n89 = Bundle By Name(cluster=w290, "Horizontal"=w300) -> (w304:cluster{"Horizontal":i16, "Vertical":i16})
        n90 = Bundle By Name(cluster=w290, "Horizontal"=i16 310, "Vertical"=w297) -> (w303:cluster{"Horizontal":i16, "Vertical":i16})
        n91 = global read "Material-Application-Constants.vi" "Color.Selection"() -> (w287:u32)
        n92 = Add(x=cluster{"Horizontal":i16, "Vertical":i16} {"Horizontal"=24, "Vertical"=0}, y=w290) -> (x+y=w288:cluster{"Horizontal":i16, "Vertical":i16})
        n93 = Unbundle By Name(w288) -> ("Horizontal"=w301:i16, "Vertical"=w298:i16)
        n94 = property on="UserInterface-Pane-Page" class="Pane"(error in=w305, "Minimum Pane Size"=w288) -> (error out=w312:errorcluster)  [unwired: 1 in, 1 out]
        n95 = property on="UserInterface-Pane-Navigation" class="Pane"("Minimum Pane Size"=w304) -> (error out=w310:errorcluster)  [unwired: 2 in, 1 out]
        n96 = property on="UserInterface-Pane-Buttons" class="Pane"("Minimum Pane Size"=w303) -> (error out=w309:errorcluster)  [unwired: 2 in, 1 out]
        n97 = property on="UI_Tree_Navigation" class="Tree (strict)"(error in=w291, "Value"="", "SelMode"=1 ("Selection Mode"), "ActiveColNum"=0 ("Active Cell:Active Column Number"), "Width"=w306, "SelColor"=w287) -> (error out=w286:errorcluster)  [unwired: 1 in, 1 out]
        n98 = Add(x=w300, y=w301) -> (x+y=w299:i16)
        n99 = Add(x=w297, y=w298) -> (x+y=w296:i16)
        n100 = Bundle By Name(cluster=cluster{"Height":i16, "Width":i16} {"Height"=0, "Width"=0} ("Size"), "Height"=w296, "Width"=w299) -> (w284:cluster{"Height":i16, "Width":i16})
        n101 = Merge Errors(w286, w312, w310, w309) -> (w311:errorcluster)
        n102 = Add(x=cluster{"Height":i16, "Width":i16} {"Height"=2, "Width"=2} ("Size"), y=w284) -> (x+y=w283:cluster{"Height":i16, "Width":i16})
        n103 = invoke class="VI" method="FP.Run-Time Position.Centered"(error in=w311, "Monitor"=w283) -> (error out=w294:errorcluster)  [unwired: 3 in, 4 out]
      }
      frame "Framework: UI Ready" {
        n104 = control-ref of="?"() -> (w317:refnum<vi>)
        n105 = call "FTW-Panel-FrontPanel-Open.vi"("error in"=w319, "VI Ref"=w317) -> ("error out"=w318:errorcluster)  [unwired: 8 in, 1 out]
      }
      frame "FTW: Error Handler" {
        w325 = T6 2 items=["no dialog", "OK message", "continue or stop message", "OK message + warnings", "continue/stop + warnings"] ("type of dialog (OK msg:1)")
        n106 = call <vilib>:"Simple Error Handler.vi"("type of dialog (OK msg:1)"=w325, "error in (no error)"=w324) -> ("error out"=w323:errorcluster)  [unwired: 3 in, 4 out]
        n107 = call "FTW-ERR-SerializeForLog.vi"("error in"=w323) -> ()  [unwired: 1 out]
        n108 = call "FTW-ERR-NoErrorConstant.vi"() -> ("no error"=w326:errorcluster)
      }
      frame "FTW: Unknown Job", Default {
        n109 = call "FTW-ERR-UnknownJob.vi"("error in"=w333, "Unknown Job"=w330) -> ("error out"=w332:errorcluster)  [unwired: 9 in]
      }
      frame "Framework: Shutdown" {
        n110 = control-ref of="?"() -> (w347:refnum<vi>)
        n111 = call "FTW-Panel-FrontPanel-Hide.vi"("error in"=w348, "VI Ref"=w347) -> ("error out"=w338:errorcluster)  [unwired: 8 in, 1 out]
        n112 = Unbundle By Name(w337) -> ("Update Service"=w339:refnum<class "Deploy-UpdateService.lvclass">)
        n113 = call <resource>:"Deploy-UpdateService-Stop.vi"("Update Service"=w339, "error in"=w338) -> ("error out"=w336:errorcluster)  [unwired: 13 in]
        n114 = call "Material-ConfigDialog-BroadcastMessage.vi"("Configuration Dialog"=w337, "Parameter"="PageCommand: Shutdown", "error in"=w336) -> ("Configuration Dialog out"=w340:refnum<class "Material-ConfigDialog.lvclass">, "error out"=w349:errorcluster)  [unwired: 11 in]
        n115 = call "Material-ConfigDialog-Destroy.vi"("Configuration Dialog"=w340, "error in"=w349) -> ()  [unwired: 13 in, 1 out]
        n116 = call <instrlib>:"Close.vi"() -> ("error out"=w344:errorcluster)  [unwired: 11 in]
        n117 = Unbundle(w346) -> ("Configuration Dialog Mailbox"=w345:refnum<event-registration>, "Update Service Event Registration"=w343:refnum<event-registration>)
        n118 = Unregister For Events(event registration refnum=w345) -> (error out=w342:errorcluster)  [unwired: 1 in]
        n119 = Unregister For Events(event registration refnum=w343) -> (error out=w341:errorcluster)  [unwired: 1 in]
        n120 = Merge Errors(w342, w341, w344) -> (w352:errorcluster)
      }
      frame "Framework: Exit" {
        n121 = control-ref of="?"() -> (w355:refnum<vi>)
        n122 = call "FTW-Panel-FrontPanel-Close.vi"("error in"=w354, "VI Ref"=w355) -> ("error out"=w353:errorcluster)  [unwired: 8 in, 1 out]
      }
      frame "--------- Sequences ---------" {
      }
      frame "Sequence: Shutdown" {
        w366 = "Framework: Shutdown\nFramework: Exit"  # Application Shutdown
        n123 = call "FTW-SEQ-AddNext.vi"("Add Next in Sequence"=w366, "Sequencer"=w364) -> ("Sequencer out"=w369:refnum<class "FTW-Sequencer.lvclass">)  [unwired: 2 in]
      }
      frame "Sequence: Check For Update" {
        n124 = in-place {
          in-place-border: w373 -> [w380]
          in-place-border: [w378] -> w372
          n125 = in-place-cluster #5(w371) -> ("Update Service"=w382:refnum<class "Deploy-UpdateService.lvclass">, "Version"=w379:string)  [unwired: 1 out]
          n126 = Equal?(x=w379, y="IDE") -> (x = y?=w376:bool)
          n127 = case shown="False" w376 {
            tunnel: [w387 w390] -> w383
            tunnel: [w386 w389] -> w378
            tunnel: w382 -> [w385 w390]
            tunnel: w380 -> [w384 w389]
            frame False {
              n128 = call <resource>:"Deploy-UpdateService-CheckNow.vi"("Update Service"=w385, "Show UI?"=FALSE, "error in"=w384) -> ("Update Service out"=w387:refnum<class "Deploy-UpdateService.lvclass">, "error out"=w386:errorcluster)  [unwired: 11 in]
            }
            frame True {
            }
          }
          n129 = in-place-cluster #5("User Menu Update Check"=FALSE, "Update Service"=w383, "Version"=w379) -> (w370:refnum<class "Material-ConfigDialog.lvclass">)
        }
      }
      frame "--------- Application Logic ---------" {
      }
      frame "UI: Shutdown Requested" {
        w396 = TRUE  # Shutdown Conditionally Allowed?
        n130 = case shown="True" w396 {
          tunnel: [w403 w407] -> w398
          tunnel: "Sequence: Shutdown" ("Add to Top of Queue") -> [w403 w405]
          frame False {
          }
          frame True {
            w406 = ""  # Do nothing... return to dialog without shutting down.
            n131 = Two Button Dialog(message="Are you sure you want to shut down?", 1:"Shutdown now" ("F button name (\"Cancel\")"), 2:"Not yet" ("T button name (\"OK\")")) -> (T button?=w408:bool)
            n132 = Select(t=w406, s=w408, f=w405) -> (s? t:f=w407:string)
          }
        }
        n133 = call "FTW-SEQ-AddNext.vi"("Add Next in Sequence"=w398, "Sequencer"=w399) -> ("Sequencer out"=w401:refnum<class "FTW-Sequencer.lvclass">)  [unwired: 2 in]
      }
      frame "UI: Set Front Panel Title" {
        n134 = disable-structure shown="Enabled" {
          frame Disabled {
            w415 = FALSE  # Show Dirty Dot?
            n135 = Select(t="Deployment Configuration*", s=w415, f="Deployment Configuration") -> (s? t:f=w418:string)
            n136 = property class="VI"("Front Panel.Title"=w418) -> ()  [unwired: 2 in, 2 out]
          }
          frame Enabled {
          }
        }
      }
      frame "Pages: Discover" {
        w425 = FALSE  # Collapse all new items?
        w428 = TRUE  # Delete Tree Items First?
        # "Make it go to the default page; in the future,\nthis can be replaced by a \"Last Page Visited\""
        n137 = call "Material-ConfigDialog-DiscoverPages.vi"("Custom Config Pages Directory"=path "", "error in"=w420) -> ("Display Names"=w423:string[], "Tree Tags"=w424:string[], "error out"=w422:errorcluster)  [unwired: 9 in, 2 out]
        n138 = for {
          tunnel: T3 {"Tag"="", "Parent"="", "Add to Top of Parent"=FALSE, "Type"="", "Indent"=0, "Child Only"=FALSE, "First Cell"="", "Next Cells"=[]} -> [w440]
          tunnel: [w439] -> w426 mode=indexing
          tunnel: w424 -> [w436] mode=indexing
          tunnel: w423 -> [w438] mode=indexing
          n139 = Bundle By Name(cluster=w440, "Child Only"=TRUE, "First Cell"=w438, "Tag"=w436) -> (w439:T3)
        }
        n140 = control-ref of="UI_Tree_Navigation"() -> (w430:refnum<vi>)
        n141 = call "Material-Glue-Tree-AddItems.vi"("Tree Ctl Ref"=w430, "Tree Items to Create"=w426, "Delete Tree Items First?"=w428, "Collapse all new items?"=w425, "error in"=w422) -> ("error out"=w429:errorcluster)  [unwired: 8 in, 2 out]
        n142 = Index Array(array=w424, index=0) -> (element=w431:string)
        n143 = property on="UI_Tree_Navigation" class="Tree (strict)"(error in=w429, "Val(Sgnl)"=w431) -> (error out=w432:errorcluster)  [unwired: 1 in, 1 out]
      }
      frame "Pages: Save" {
        n144 = local read "UI_Tree_Navigation"() -> (w444:string)
        n145 = call "Material-ConfigDialog-MessageToPageID.vi"("Configuration Dialog"=w442, "Parameter"="PageCommand: Settings Saved", "PageID"=w444, "error in"=w441) -> ("Configuration Dialog out"=w446:refnum<class "Material-ConfigDialog.lvclass">, "error out"=w445:errorcluster)  [unwired: 10 in]
      }
      frame "Pages: Revert" {
        n146 = local read "UI_Tree_Navigation"() -> (w452:string)
        n147 = call "Material-ConfigDialog-MessageToPageID.vi"("Configuration Dialog"=w450, "Parameter"="PageCommand: Revert", "PageID"=w452, "error in"=w449) -> ("Configuration Dialog out"=w453:refnum<class "Material-ConfigDialog.lvclass">, "error out"=w454:errorcluster)  [unwired: 10 in]
      }
    }
  }
  "error out" <- w4
  n148 = call "FTW-SEQ-Destroy.vi"("Sequencer"=w1) -> ()  [unwired: 1 in]
